vi "SR830 DS345 Set OF and Read Single.vi"(0 "Lock-in GPIB address":string="0:9", 5 "SRS DS345 GPIB address":string="0:19", 7 "Oscillator Frequency (Hz)":dbl=1126.0 min=0.001 max=250000.0 step=0.001 format="%.3f", 9 "Wait Time (sec)":dbl=0.1 min=0.001 max=250000.0 step=0.001 format="%.3f", 11 "error in":T1) -> (6 "f,x1,y1,aux11,aux12":dbl[](array[numeric]), 15 "error out":errorcluster)   [LabVIEW 2015]
panel:
  out "Freq. (Hz)":dbl=699.3822116409185 format="%.2f"
  out "Y1":dbl=0.999751876482715 format="%.2f"
  out "X1":dbl=0.999751876482715 format="%.2f"
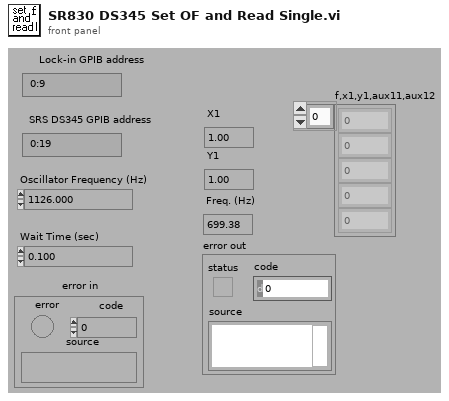
[diagram p1: front panel]
types:
  T1 = cluster{"error":bool, "code":i32, "source":string}
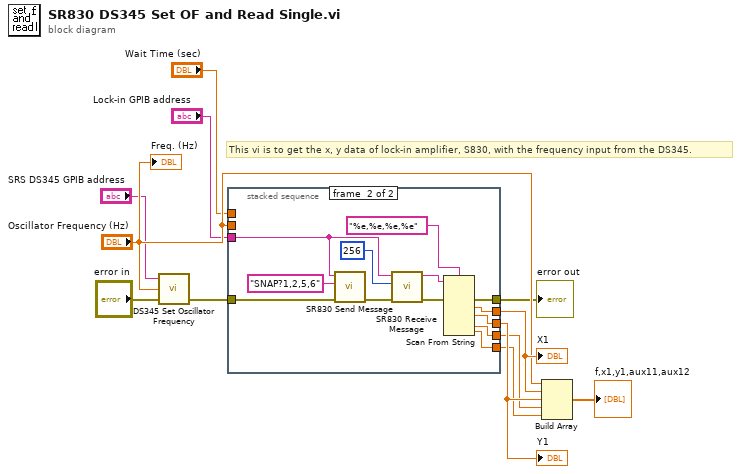
[diagram p0: block diagram]
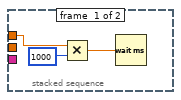
[diagram p2: hidden frame]
diagram:
  # "This vi is to get the x, y data of lock-in amplifier, S830, with the frequency input from the DS345."
  n1 = call "DS345 Set Oscillator Frequency.vi"("error in"="error in", "Freq. (Hz)"="Oscillator Frequency (Hz)", "GPIB address"="SRS DS345 GPIB address") -> ("error out"=w11:T1)  [unwired: 2 out]
  n2 = stacked-sequence {
    tunnel: [_ w21] -> w10
    tunnel: [_ w20] -> w9
    tunnel: "Lock-in GPIB address" -> [_ w22]
    tunnel: w11 -> [_ w16]
    tunnel: "Oscillator Frequency (Hz)" -> [_ _]
    tunnel: [_ w19] -> w6
    tunnel: [_ w18] -> w5
    tunnel: [_ w17] -> w7
    tunnel: "Wait Time (sec)" -> [w13 _]
    frame #0 {
      n3 = Multiply(x=w13, y=i16 1000) -> (x*y=w15:dbl)
      n4 = Wait (ms)(milliseconds to wait=w15) -> ()  [unwired: 1 out]
    }
    frame #1 {
      n5 = call "SR830 Send Message.vi"("address string"=w22, "write buffer"="SNAP?1,2,5,6", "error in"=w16) -> ("error out"=w27:T1)  [unwired: 3 in, 3 out]
      n6 = call "SR830 Receive Message.vi"("address string"=w22, "byte count"=256, "error in"=w27) -> ("read buffer"=w24:string, "error out"=w25:T1)  [unwired: 3 in, 2 out]
      n7 = Scan From String(format string="%e,%e,%e,%e", input string=w24, error in=w25) -> (error out=w17:errorcluster, output 1=w21:dbl, output 2=w20:dbl, output 3=w19:dbl, output 4=w18:dbl)  [unwired: 1 in, 6 out]
    }
  }
  "X1" <- w10
  "Y1" <- w9
  "error out" <- w7
  n8 = Build Array("Oscillator Frequency (Hz)", w10, w9, w6, w5) -> (→"f,x1,y1,aux11,aux12":dbl[])
  "Freq. (Hz)" <- "Oscillator Frequency (Hz)"
